vi "MM9.ChangeFilePrefix.vi"(0 "i ref in":refnum<vi>, 2 "filePrefix":string, 3 "ms timeout (10000)":i32=10000, 5 "error in (no error)":errorcluster) -> (14 "i ref out":refnum<vi>, 17 "timed out":bool, 19 "error out":errorcluster)   [LabVIEW 2014, in "MM9.lvlib"]
doc: "Changes the file prefix of the disc archiver."
uses:
  MM9.lvlib
  CS_Core/CSSystem/CoreLib/CoreLib.string 2 byte array.vi
  CS_Core/CSSystem/CoreLib/CoreLib.lvlib
  CS_Core/BaseProcess/BaseProcess.lvlib
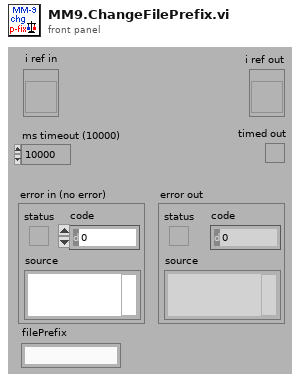
[diagram p1: front panel]
types:
  T1 = typedef "CoreDefs.rawDataType.ctl" = i8[]
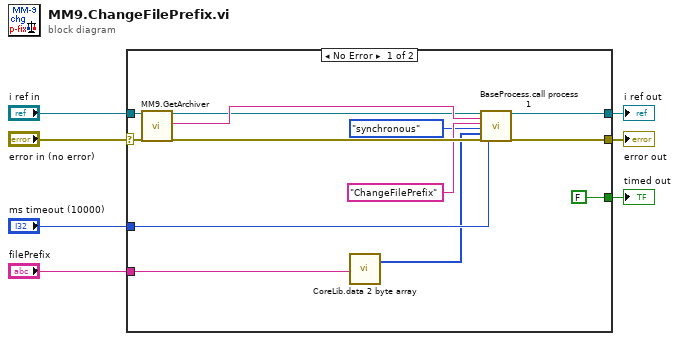
[diagram p0: block diagram]
diagram:
  n1 = case shown="No Error" "error in (no error)" {
    selector: "error in (no error)" -> [w12 w21]
    tunnel: [FALSE ("timed out") _] -> w7
    tunnel: [w18 w22] -> w6
    tunnel: [w17 w21] -> w5
    tunnel: "i ref in" -> [w14 w22]
    tunnel: "ms timeout (10000)" -> [w13 _]
    tunnel: "filePrefix" -> [w11 _]
    frame No Error {
      n2 = call "MM9.GetArchiver.vi"("i ref in"=w14, "error in (no error)"=w12) -> ("i ref out"=w16:refnum<vi>, "archiver"=w19:string, "error out"=w15:errorcluster)  [unwired: 15 in]
      n3 = call-poly "CoreLib.data 2 byte array.vi"("string"=w11) -> ("byteArray out"=w8:T1)  [unwired: 18 in]
      n4 = call "BaseProcess.call process 1.vi"("i ref in"=w16, "Object"=w19, "Selector"="ChangeFilePrefix", "CallType"=enum16{"simple", "synchronous", "asynchronous"}."synchronous", "Data"=w8, "error in (no error)"=w15, "timeout (ms)"=w13) -> ("i ref out"=w18:refnum<vi>, "error out"=w17:errorcluster)  [unwired: 10 in, 1 out]
    }
    frame Error {
    }
  }
  "error out" <- w5
  "i ref out" <- w6
  "timed out" <- w7
